vi "Cpp-Solver.vi"(10 "Word List":string[](array[string]), 11 "Word Search Grid":string[][](array[string])) -> (3 "Solutions":T1)   [LabVIEW 2020]
uses:
  support/Solutions--map.ctl
  support/Letter Index--cluster.ctl
  wss.64.dll
panel:
  # "Implement your Word Search challenge solution in this VI. Do not change the connector pane of this VI."
  # "Letters will always be ALL CAPS."
  # "Words will always be ALL CAPS."
  # "The Word Search Grid contains the 2D array of letters in which all words in the Word List appear. Words can appear forwards, backwards, up, down, and diagonally in any direction.\n\nThe Solutions map will contain one entry per item in the Word List. The map elements are:\n\nWord: The word from the Word List.\nLetter Indices: The row/column indices into the Word Search Grid for each letter (in order) in the word."
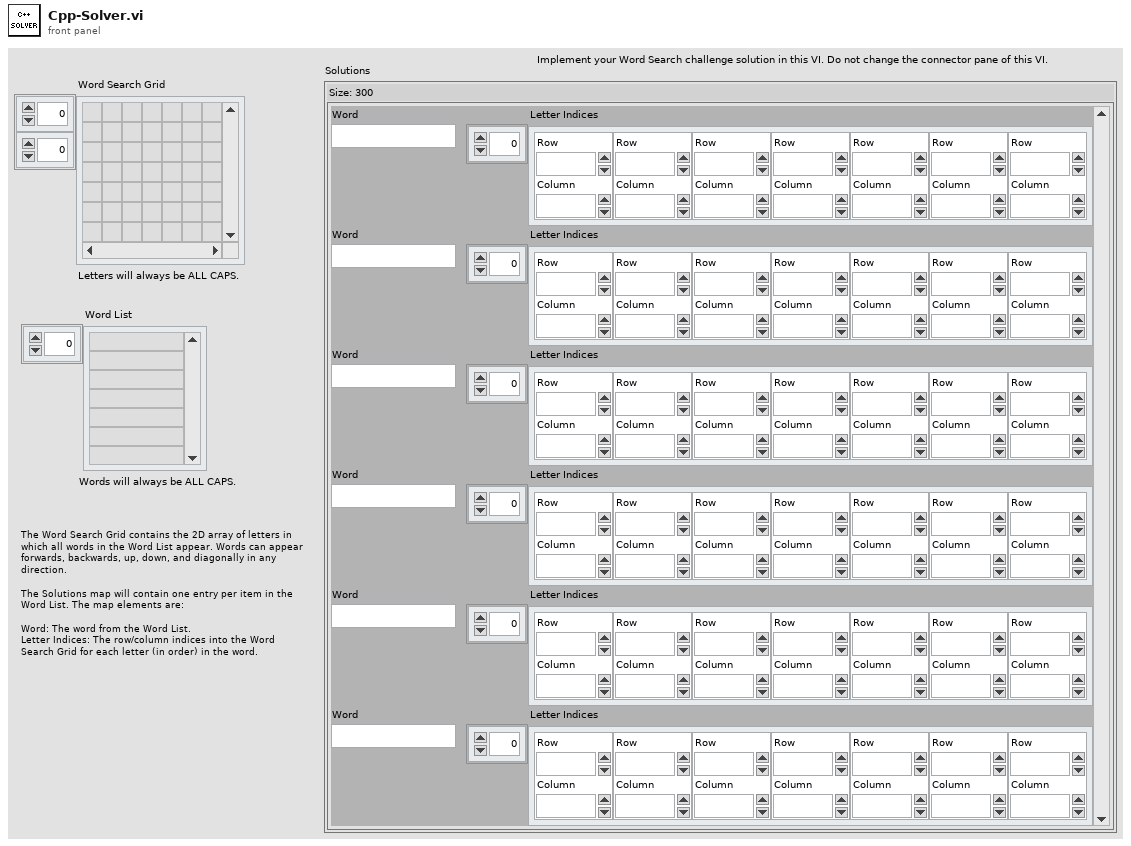
[diagram p1: front panel]
types:
  T1 = typedef "Solutions--map.ctl" = map{string, T2[]}
  T2 = typedef "Letter Index--cluster.ctl" = cluster{"Row":i32, "Column":i32}
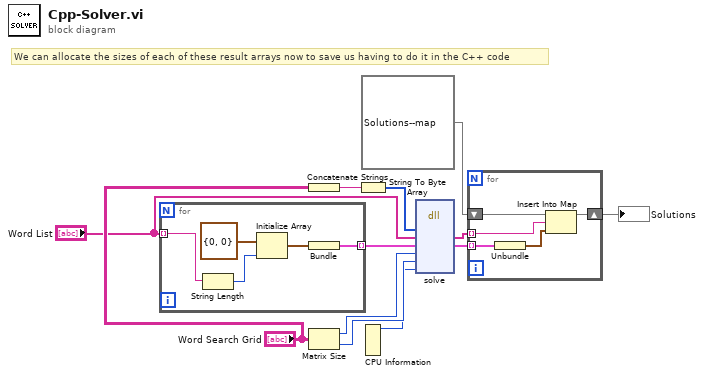
[diagram p0: block diagram]
diagram:
  # "We can allocate the sizes of each of these result arrays now to save us having to do it in the C++ code"
  n1 = for {
    tunnel: "Word List" -> [w17] mode=indexing
    tunnel: [w13] -> w8 mode=indexing
    n2 = String Length(string=w17) -> (length=w15:i32)
    n3 = Initialize Array(T2 {"Row"=0, "Column"=0} ("Letter Index"), w15) -> (w14:T2[])
    n4 = Bundle(w14) -> (w13:cluster{T2[]})  [unwired: 1 in]
  }
  n5 = Concatenate Strings("Word Search Grid") -> (w12:string)
  n6 = Matrix Size(0:"Word Search Grid") -> (1:w7:i32, 2:w6:i32)
  n7 = String To Byte Array(string=w12) -> (unsigned byte array=w10:u8[])
  n8 = CPU Information() -> (4:w1:i32)  [unwired: 3 out]
  n9 = dll-call lib="D:/sol-2024-word-search-main/sol-2024-word-search-main/wss.*.*" fn="solve"("board_pointer"=w10, "word_list"="Word List", "results"=w8, "board_rows"=w7, "board_cols"=w6, "n_threads"=w1) -> ("word_list"=w4:string[], "results"=w5:cluster{T2[]}[])  [unwired: 8 in, 2 out]
  n10 = for {
    tunnel: w5 -> [w21] mode=indexing
    tunnel: w4 -> [w22] mode=indexing
    shift-right: [w19] -> w2
    shift-left: T1 {} ("Solutions") -> [w20]
    n11 = Unbundle(w21) -> (w18:T2[])
    n12 = Insert Into Map(map in=w20, key=w22, value=w18) -> (map out=w19:T1)  [unwired: 2 out]
  }
  "Solutions" <- w2
